vi "main.vi"() -> ()   [LabVIEW 2017]
uses:
  <vilib>/DAQmx/read.llb/DAQmx Read (Analog 1D DBL NChan 1Samp).vi
  <vilib>/DAQmx/configure/timing.llb/DAQmx Timing (Sample Clock).vi
  <vilib>/DAQmx/miscellaneous.llb/DAQmx Fill In Error Info.vi
panel:
  in  "Scale b":dbl[](array[numeric])
  in  "Scale a":dbl[](array[numeric])
  out "drehmoment_kraft":dbl[][](graph)
  out "temperature":dbl[][](graph)
  in  "stop":bool
  # "y = a * x + b"
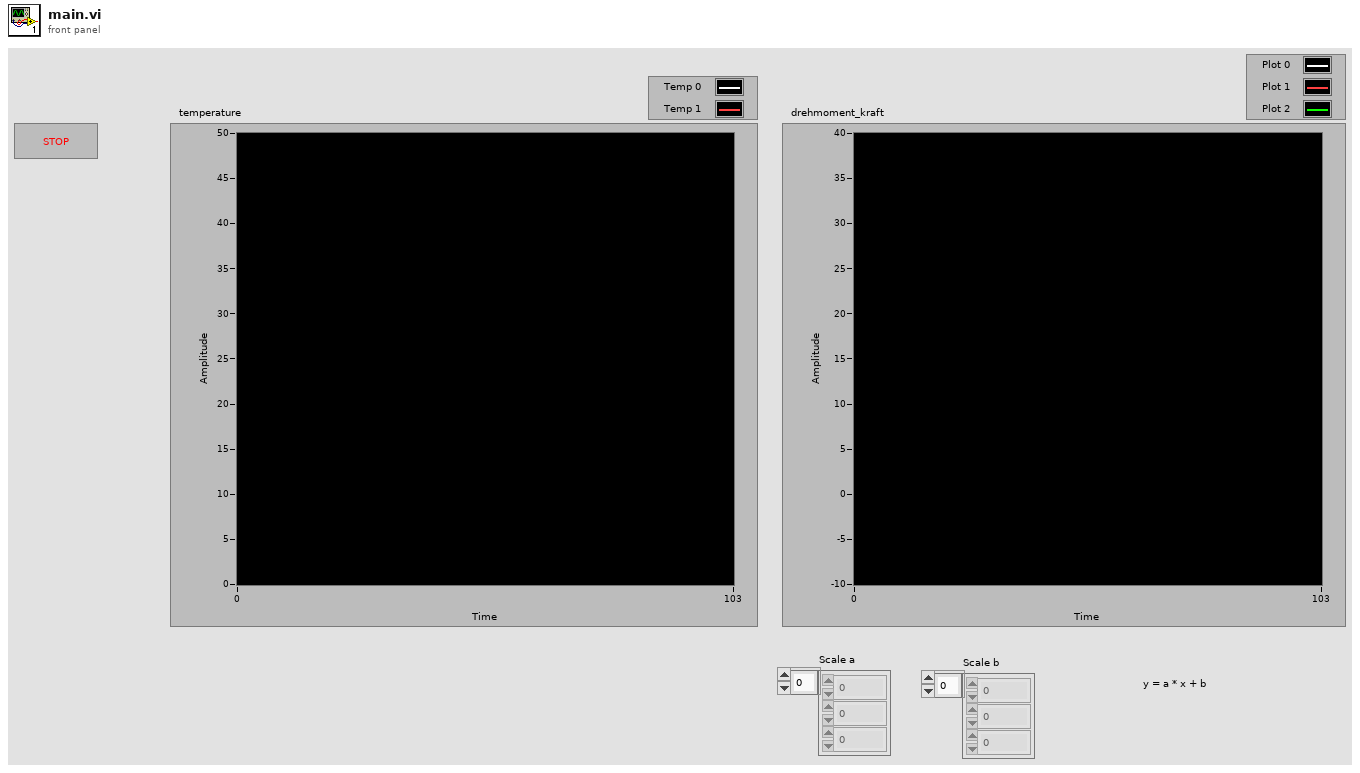
[diagram p1: front panel]
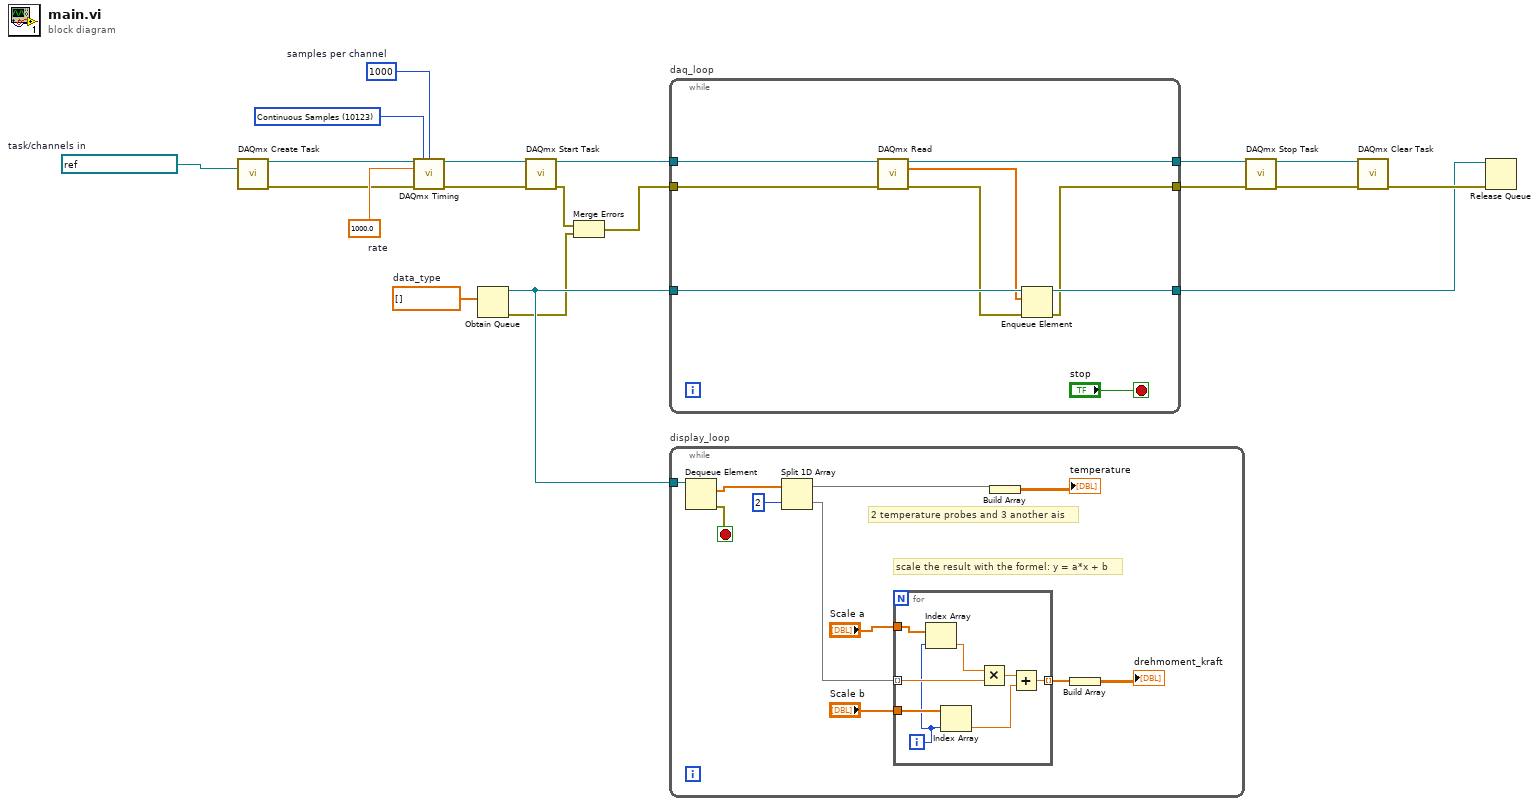
[diagram p0: block diagram]
diagram:
  w13 = dbl[] []  # data_type
  w18 = 1000.0  # rate
  w19 = 1000  # samples per channel
  w20 = 10123 items=["Finite Samples"=10178, "Continuous Samples"=10123, "Hardware Timed Single Point"=12522] ("sample mode")
  w5 = refnum<k21> "AnalogReadTask"  # task/channels in
  n1 = call <vilib>:"DAQmx Create Task.vi"("task to copy"=w5) -> ("task out"=w6:refnum<k21>, "error out"=w7:errorcluster)  [unwired: 13 in]
  n2 = call-poly <vilib>:"DAQmx Timing.vi"("task/channels in"=w6, "sample mode"=w20, "samples per channel"=w19, "rate"=w18, "error in"=w7) -> ("task out"=w2:refnum<k21>, "error out"=w1:errorcluster)  [unwired: 9 in]
  n3 = Obtain Queue(element data type=w13) -> (queue out=w12:refnum<queue>, error out=w9:errorcluster)  [unwired: 4 in, 1 out]
  n4 = call <vilib>:"DAQmx Start Task.vi"("task/channels in"=w2, "error in"=w1) -> ("task out"=w4:refnum<k21>, "error out"=w3:errorcluster)  [unwired: 12 in]
  n5 = Merge Errors(w3, w9) -> (w14:errorcluster)
  n6 = while "daq_loop" {
    tunnel: w14 -> [w28]
    tunnel: w4 -> [w27]
    tunnel: [w26] -> w17
    tunnel: w12 -> [w25]
    tunnel: [w24] -> w10
    tunnel: [w22] -> w8
    stop <- "stop" stop-if-true
    n7 = call-poly <vilib>:"DAQmx Read.vi"("task/channels in"=w27, "error in"=w28) -> ("task out"=w26:refnum<k21>, "data"=w21:dbl[], "error out"=w23:errorcluster)  [unwired: 11 in]
    n8 = Enqueue Element(queue=w25, element=w21, error in (no error)=w23) -> (queue out=w24:refnum<queue>, error out=w22:errorcluster)  [unwired: 1 in, 1 out]
  }
  n9 = while "display_loop" {
    tunnel: w12 -> [w40]
    stop <- w39 stop-if-true
    # "2 temperature probes and 3 another ais"
    # "scale the result with the formel: y = a*x + b"
    n10 = Dequeue Element(queue=w40) -> (element=w38:dbl[], error out=w39:errorcluster)  [unwired: 2 in, 2 out]
    n11 = Split 1D Array(array=w38, index=2) -> (first subarray=w36:dbl[], second subarray=w34:dbl[])
    n12 = for {
      tunnel: w34 -> [w48] mode=indexing
      tunnel: "Scale a" -> [w44]
      tunnel: "Scale b" -> [w43]
      tunnel: [w46] -> w31 mode=indexing
      i -> [w42]
      n13 = Index Array(array=w44, index=w42) -> (element=w45:dbl)
      n14 = Index Array(array=w43, index=w42) -> (element=w41:dbl)
      n15 = Multiply(x=w45, y=w48) -> (x*y=w47:dbl)
      n16 = Add(x=w47, y=w41) -> (x+y=w46:dbl)
    }
    n17 = Build Array(w36) -> (→"temperature":dbl[][])
    n18 = Build Array(w31) -> (→"drehmoment_kraft":dbl[][])
  }
  n19 = call <vilib>:"DAQmx Stop Task.vi"("task/channels in"=w17, "error in"=w8) -> ("task out"=w15:refnum<k21>, "error out"=w16:errorcluster)  [unwired: 12 in]
  n20 = call <vilib>:"DAQmx Clear Task.vi"("task in"=w15, "error in"=w16) -> ("error out"=w11:errorcluster)  [unwired: 13 in]
  n21 = Release Queue(queue=w10, error in (no error)=w11) -> ()  [unwired: 1 in, 3 out]
